vi "Read_Write INI File.vi"(5 "Mode":enum16{"Read", "Write"}(ring), 6 "Indicators too?":bool, 7 "Section":string, 8 "error in":errorcluster, 9 "Filepath":path, 11 "Ctl Refnum":refnum<vi>[](array[refnum])) -> (0 "error out":errorcluster)   [LabVIEW 2020]
uses:
  <vilib>/Utility/config.llb/NI_LVConfig.lvlib
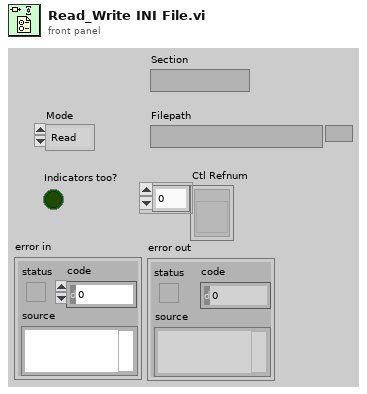
[diagram p1: front panel]
types:
  T1 = typedef "NI_LVConfig.lvlib/Config Data RefNum.ctl" = refnum<k1>
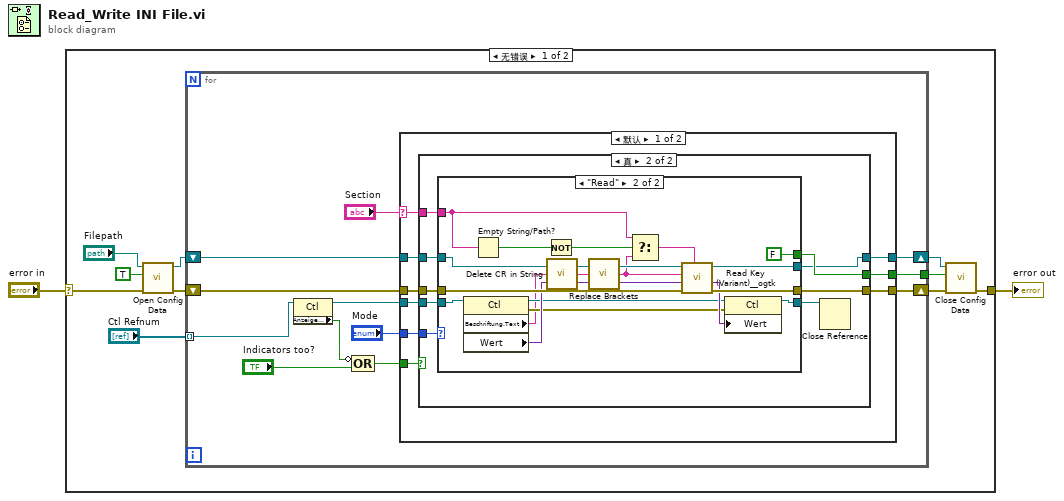
[diagram p0: block diagram]
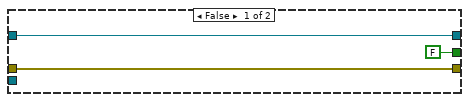
[diagram p2: hidden frame]
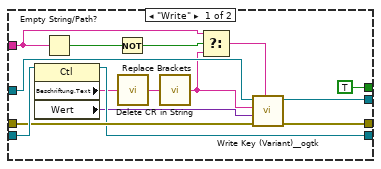
[diagram p3: hidden frame]
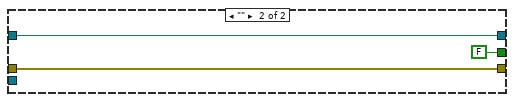
[diagram p4: hidden frame]
diagram:
  n1 = case shown="无错误" "error in" {
    selector: "error in" -> [w6 w82]
    tunnel: [w8 w82] -> w1
    frame No Error {
      n2 = call <vilib>:"Open Config Data.vi"("error in (no error)"=w6, "create file if necessary (T)"=TRUE ("create file if necessary? (T)"), "configuration file path"="Filepath") -> ("error out"=w5:errorcluster, "refnum"=w3:T1)  [unwired: 6 in, 1 out]
      n3 = for {
        tunnel: "Ctl Refnum" -> [w22] mode=indexing
        tunnel: [w16] -> w10
        shift-right: [w17] -> w11
        shift-left: w5 -> [w14]
        shift-right: [w15] -> w9
        shift-left: w3 -> [w13]
        n4 = property class="Ctl"(reference=w22) -> (reference out=w23:refnum<vi>, "Anzeigeelement"=w21:bool)  [unwired: 1 in, 1 out]
        n5 = Compound Arithmetic op=OR(invert w21, "Indicators too?") -> (w19:bool)
        n6 = case shown="默认" "Section" {
          selector: "Section" -> [w28 _]
          tunnel: "Mode" -> [w33 _]
          tunnel: w13 -> [w32 w80]
          tunnel: w14 -> [w31 w81]
          tunnel: w23 -> [w30 _]
          tunnel: w19 -> [w29 _]
          tunnel: [w27 w81] -> w17
          tunnel: [w26 FALSE ("write configuration file? (F)")] -> w16
          tunnel: [w25 w80] -> w15
          frame Default {
            n7 = case shown="真" w29 {
              tunnel: w28 -> [_ w45]
              tunnel: w33 -> [_ w44]
              tunnel: w32 -> [w35 w43]
              tunnel: w31 -> [w36 w42]
              tunnel: w30 -> [_ w40]
              tunnel: [w36 w39] -> w27
              tunnel: [FALSE ("write configuration file? (F)") w38] -> w26
              tunnel: [w35 w37] -> w25
              frame False {
              }
              frame True {
                n8 = case shown="\"Read\"" w44 {
                  tunnel: [w47 w67] -> w37
                  tunnel: [w48 w72] -> w39
                  tunnel: w45 -> [w51 w62]
                  tunnel: w42 -> [w58 w75]
                  tunnel: w40 -> [w60 w78]
                  tunnel: [TRUE ("write configuration file? (F)") FALSE ("write configuration file? (F)")] -> w38
                  tunnel: w43 -> [w57 w76]
                  tunnel: [w55 w73] -> w41
                  frame "Write" {
                    n9 = property class="Ctl"(reference=w60) -> (reference out=w55:refnum<vi>, "Beschriftung.Text"=w54:string, "Wert"=w50:variant)  [unwired: 1 in, 1 out]
                    n10 = Empty String/Path?(string/path=w51) -> (empty?=w53:bool)
                    n11 = Not(x=w53) -> (.not. x?=w52:bool)
                    n12 = call "Delete CR in String.vi"("Input String"=w54) -> ("String without CR"=w56:string)  [unwired: 4 out]
                    n13 = call "Replace Brackets.vi"("Label.Text"=w56) -> ("String"=w46:string)  [unwired: 4 out]
                    n14 = Select(t=w51, s=w52, f=w46) -> (s? t:f=w49:string)
                    n15 = call "Write Key (Variant)__ogtk.vi"("section"=w49, "error in (no error)"=w58, "key-value"=w50, "key (optional)"=w46, "refnum"=w57) -> ("error out"=w48:errorcluster, "refnum out"=w47:T1)  [unwired: 5 in]
                  }
                  frame "Read" {
                    n16 = property class="Ctl"(reference=w78) -> (reference out=w68:refnum<vi>, error out=w69:errorcluster, "Beschriftung.Text"=w66:string, "Wert"=w70:variant)  [unwired: 1 in]
                    n17 = Empty String/Path?(string/path=w62) -> (empty?=w65:bool)
                    n18 = Not(x=w65) -> (.not. x?=w64:bool)
                    n19 = call "Delete CR in String.vi"("Input String"=w66) -> ("String without CR"=w74:string)  [unwired: 4 in]
                    n20 = call "Replace Brackets.vi"("Label.Text"=w74) -> ("String"=w61:string)  [unwired: 4 in]
                    n21 = Select(t=w62, s=w64, f=w61) -> (s? t:f=w63:string)
                    n22 = call "Read Key (Variant)__ogtk.vi"("section"=w63, "error in (no error)"=w75, "type"=w70, "key (optional)"=w61, "refnum"=w76) -> ("error out"=w72:errorcluster, "key-value"=w71:variant, "refnum out"=w67:T1)  [unwired: 3 in, 1 out]
                    n23 = property class="Ctl"(reference=w68, error in=w69, "Wert"=w71) -> (reference out=w73:refnum<vi>)  [unwired: 1 out]
                  }
                }
                n24 = Close Reference(reference=w41) -> ()  [unwired: 1 in, 1 out]
              }
            }
          }
          frame "" {
          }
        }
      }
      n25 = call <vilib>:"Close Config Data.vi"("error in (no error)"=w11, "write file if changed (T)"=w10, "refnum"=w9) -> ("error out"=w8:errorcluster)  [unwired: 7 in, 1 out]
    }
    frame Error {
    }
  }
  "error out" <- w1
